vi "create inputs for unmapped outputs.vi"(7 "module instance":string, 8 "outputs":refnum<class "TBM channel.lvclass">[](array[class]), 9 "input channels in":refnum<class "TBM channel.lvclass">[](array[class]), 10 "engine configuration in":refnum<class "engine configuration.lvclass">, 11 "TEC configuration in":refnum<class "TEC configuration.lvclass">) -> (1 "input channels out":refnum<class "TBM channel.lvclass">[](array[class]), 2 "engine configuration out":refnum<class "engine configuration.lvclass">, 3 "TEC configuration out":refnum<class "TEC configuration.lvclass">)   [LabVIEW 2013, in "TEC editor node.lvclass"]
uses:
  TEC editor node.lvclass
  <vilib>/NI/Tag Bus Module Framework/channel/TBM channel.lvclass
  <vilib>/NI/Module Execution Interface/Engine Configuration/engine configuration.lvclass
  configuration/TEC configuration.lvclass
  <vilib>/NI/Tag Bus/tag/tag descriptor.lvclass/tag descriptor.ctl
  <vilib>/NI/Tag Bus Module Framework/channel/channel classification.ctl
  <vilib>/NI/Tag Bus Module Framework/channel/TBM channel.lvclass/TBM channel.ctl
  <vilib>/NI/Tag Bus/tag/read tag name.vi
  <vilib>/NI/Tag Bus/tag/tag descriptor.lvclass
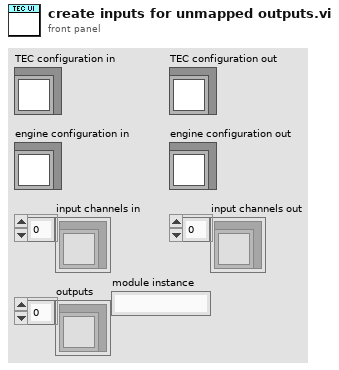
[diagram p1: front panel]
types:
  T1 = typedef "TBM channel.lvclass/channel classification.ctl" = enum16{"input data", "output data", "processing parameter", "processing result"}
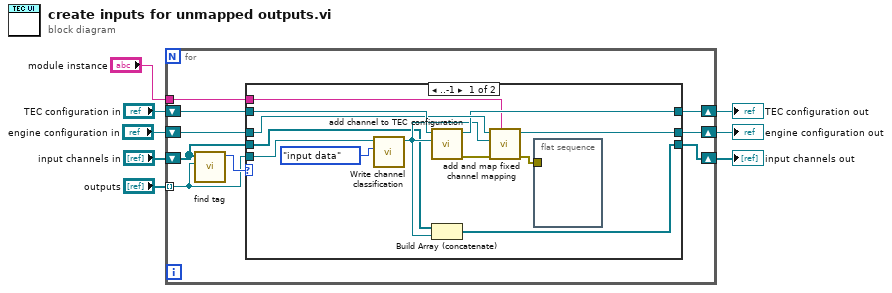
[diagram p0: block diagram]
diagram:
  n1 = for {
    shift-right: [w16] -> w6
    shift-left: "TEC configuration in" -> [w15]
    shift-right: [w12] -> w7
    shift-left: "engine configuration in" -> [w11]
    tunnel: "outputs" -> [w10] mode=indexing
    shift-right: [w13] -> w8
    shift-left: "input channels in" -> [w14]
    tunnel: "module instance" -> [w9]
    n2 = call <vilib>:"find tag.vi"("tag"=w10, "tags in"=w14) -> ("index"=w17:i32)  [unwired: 9 in]
    n3 = case shown="..-1" w17 {
      tunnel: [w23 w32] -> w16
      tunnel: w15 -> [w27 w32]
      tunnel: w14 -> [w20 w31]
      tunnel: [w19 w31] -> w13
      tunnel: [w22 w30] -> w12
      tunnel: w11 -> [w26 w30]
      tunnel: w10 -> [w29 _]
      tunnel: w9 -> [w18 _]
      frame ..-1 {
        n4 = call <vilib>:"Write channel classification.vi"("channel classification"=channel_classification."input data", "channel in"=w29) -> ("channel out"=w21:refnum<class "TBM channel.lvclass">)  [unwired: 8 in, 1 out]
        n5 = call "add channel to TEC configuration.vi"("channel"=w21, "TEC configuration in"=w27) -> ("error out"=w25:errorcluster, "TEC configuration out"=w23:refnum<class "TEC configuration.lvclass">)  [unwired: 8 in]
        n6 = Build Array (concatenate)(w20, w21) -> (w19:refnum<class "TBM channel.lvclass">[])
        n7 = call <vilib>:"add and map fixed channel mapping.vi"("module instance"=w18, "error in"=w25, "fixed channel"=w21, "engine configuration in"=w26) -> ("error out"=w24:errorcluster, "engine configuration out"=w22:refnum<class "engine configuration.lvclass">)  [unwired: 6 in]
        n8 = flat-sequence {
          tunnel: w24 -> [_]
          frame #0 {
          }
        }
      }
      frame 0.. {
        # "found, OK"
      }
    }
  }
  "input channels out" <- w8
  "engine configuration out" <- w7
  "TEC configuration out" <- w6
